vi "Test_USB.vi"(6 "VISA resource name":refnum<visa-resource-name>, 7 "Passed so far?":bool, 8 "error in (no error)":errorcluster, 11 "Slot":T1) -> (0 "error out":errorcluster, 3 "read buffer":string, 4 "VISA resource name out":refnum<visa-resource-name>, 5 "Passed?":bool)   [LabVIEW 2024]
uses:
  AP slots to test.ctl
panel:
  out "read buffer AP2":string
  out "Serial Settings:Number of Bytes at Serial Port":u32
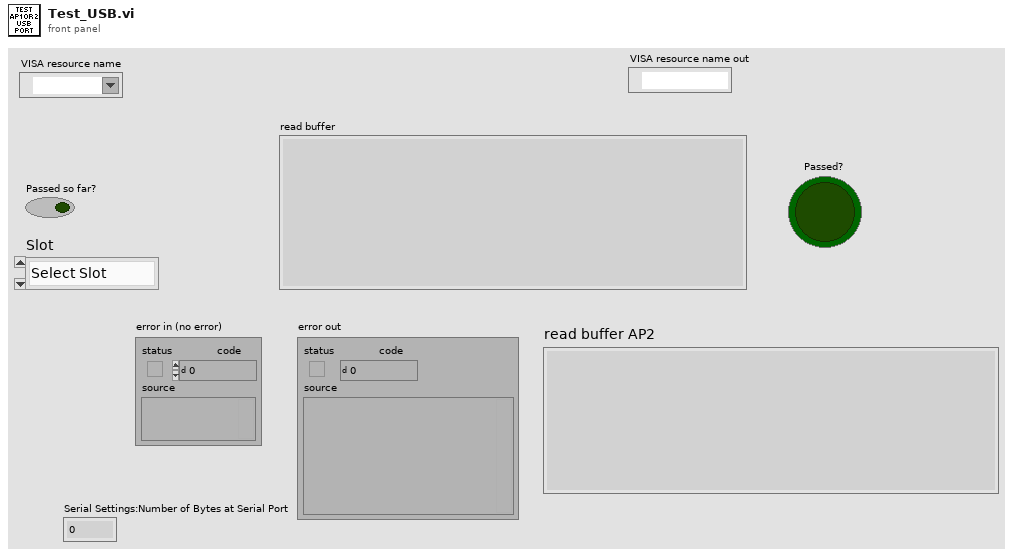
[diagram p1: front panel]
types:
  T1 = typedef "AP slots to test.ctl" = enum16{"Select Slot", "AP1", "AP2", "AP1 and AP2"}
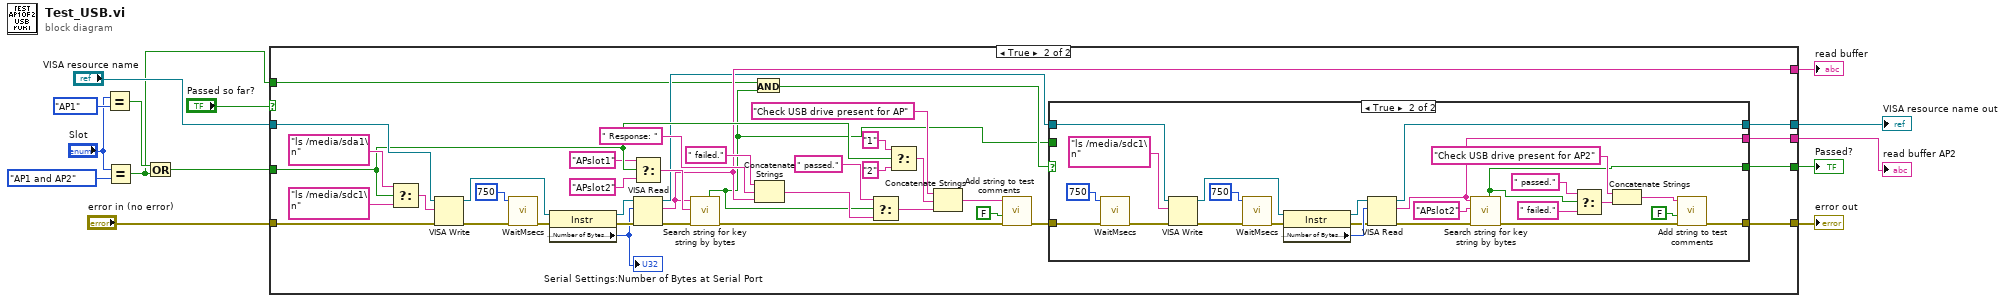
[diagram p0: block diagram]
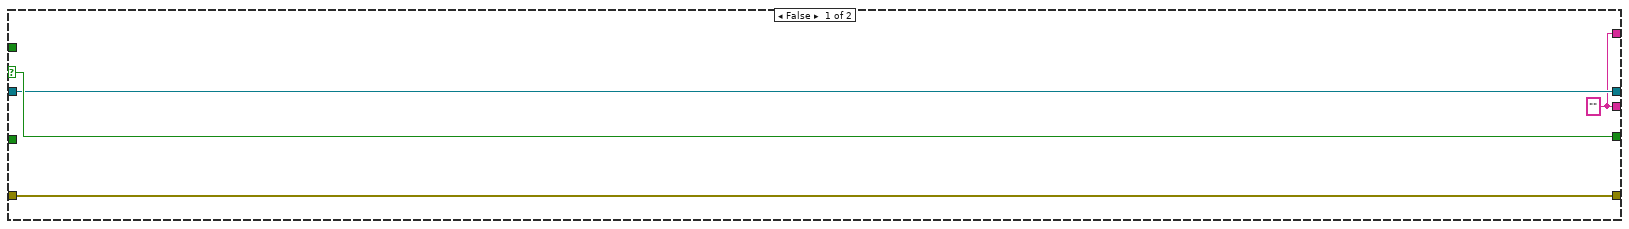
[diagram p2: hidden frame]
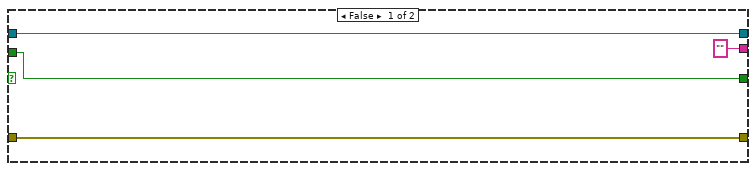
[diagram p3: hidden frame]
diagram:
  n1 = Equal?(x="Slot", y=AP_slots_to_test."AP1") -> (x = y?=w6:bool)
  n2 = Equal?(x="Slot", y=AP_slots_to_test."AP1 and AP2") -> (x = y?=w2:bool)
  n3 = Or(x=w6, y=w2) -> (x .or. y?=w5:bool)
  n4 = case shown="True" "Passed so far?" {
    selector: "Passed so far?" -> [w17 _]
    tunnel: [w18 w25] -> w14
    tunnel: w5 -> [_ w34]
    tunnel: [w17 w20] -> w13
    tunnel: "VISA resource name" -> [w16 w48]
    tunnel: [w15 w28] -> w8
    tunnel: "error in (no error)" -> [w18 w47]
    tunnel: [w16 w24] -> w9
    tunnel: w2 -> [_ w22]
    tunnel: [w15 w23] -> w1
    frame False {
      w15 = "" ("output string")
    }
    frame True {
      n5 = Select(t="ls /media/sda1\n", s=w34, f="ls /media/sdc1\n") -> (s? t:f=w51:string)
      n6 = VISA Write(VISA resource name=w48, write buffer=w51, error in (no error)=w47) -> (VISA resource name out=w49:refnum<visa-resource-name>, error out=w50:errorcluster)  [unwired: 1 out]
      n7 = call "WaitMsecs.vi"("error in (no error)"=w50, "Wait Msecs"=u32 750) -> ("error out"=w52:errorcluster)  [unwired: 9 in]
      n8 = property class="Instr"(reference=w49, error in=w52) -> (reference out=w57:refnum<visa-resource-name>, error out=w56:errorcluster, "Serial Settings:Number of Bytes at Serial Port"=w29:u32)
      "Serial Settings:Number of Bytes at Serial Port" <- w29
      n9 = Select(t="APslot1" ("Search for string"), s=w34, f="APslot2" ("Search for string")) -> (s? t:f=w31:string)
      n10 = VISA Read(VISA resource name=w57, byte count=w29, error in (no error)=w56) -> (VISA resource name out=w26:refnum<visa-resource-name>, read buffer=w28:string, error out=w35:errorcluster)  [unwired: 1 out]
      n11 = call "Search string for key string by bytes.vi"("error in (no error)"=w35, "Search for string"=w31, "String"=w28) -> ("error out"=w30:errorcluster, "Found match?"=w19:bool)  [unwired: 4 in, 3 out]
      n12 = And(x=w22, y=w19) -> (x .and. y?=w21:bool)
      n13 = Concatenate Strings(" failed.", " Response: " ("string"), w28) -> (w36:string)
      n14 = Select(t=" passed.", s=w19, f=w36) -> (s? t:f=w41:string)
      n15 = Select(t="1", s=w34, f="2") -> (s? t:f=w43:string)
      n16 = Concatenate Strings("Check USB drive present for AP" ("string"), w43, w41) -> (w40:string)
      n17 = call "Add string to test comments.vi"("error in (no error)"=w30, "New Section (y)?"=FALSE, "Comments"=w40) -> ("error out"=w27:errorcluster)  [unwired: 7 in, 1 out]
      n18 = case shown="True" w21 {
        tunnel: w27 -> [w60 w66]
        tunnel: w26 -> [w61 w83]
        tunnel: [w60 w69] -> w25
        tunnel: [w61 w68] -> w24
        tunnel: ["" ("read buffer") w62] -> w23
        tunnel: [w58 w64] -> w20
        tunnel: w19 -> [w58 _]
        frame False {
        }
        frame True {
          n19 = call "WaitMsecs.vi"("error in (no error)"=w66, "Wait Msecs"=u32 750) -> ("error out"=w65:errorcluster)  [unwired: 9 in]
          n20 = VISA Write(VISA resource name=w83, write buffer="ls /media/sdc1\n", error in (no error)=w65) -> (VISA resource name out=w82:refnum<visa-resource-name>, error out=w85:errorcluster)  [unwired: 1 out]
          n21 = call "WaitMsecs.vi"("error in (no error)"=w85, "Wait Msecs"=u32 750) -> ("error out"=w81:errorcluster)  [unwired: 9 in]
          n22 = property class="Instr"(reference=w82, error in=w81) -> (reference out=w79:refnum<visa-resource-name>, error out=w78:errorcluster, "Serial Settings:Number of Bytes at Serial Port"=w80:u32)
          n23 = VISA Read(VISA resource name=w79, byte count=w80, error in (no error)=w78) -> (VISA resource name out=w68:refnum<visa-resource-name>, read buffer=w62:string, error out=w76:errorcluster)  [unwired: 1 out]
          n24 = call "Search string for key string by bytes.vi"("error in (no error)"=w76, "Search for string"="APslot2", "String"=w62) -> ("error out"=w70:errorcluster, "Found match?"=w64:bool)  [unwired: 4 in, 3 out]
          n25 = Select(t=" passed.", s=w64, f=" failed.") -> (s? t:f=w73:string)
          n26 = Concatenate Strings("Check USB drive present for AP2" ("string"), w73) -> (w72:string)
          n27 = call "Add string to test comments.vi"("error in (no error)"=w70, "New Section (y)?"=FALSE, "Comments"=w72) -> ("error out"=w69:errorcluster)  [unwired: 7 in, 1 out]
        }
      }
    }
  }
  "error out" <- w14
  "Passed?" <- w13
  "read buffer" <- w8
  "VISA resource name out" <- w9
  "read buffer AP2" <- w1
